vi "DAC freq and lock in test.vi"() -> ()   [LabVIEW 2012]
uses:
  <vilib>/Utility/file.llb/Read From Spreadsheet File (DBL).vi
  <vilib>/express/express arith-compare/Formula/XNode/ExpressFormulaBlockNode.xnode
panel:
  in  "resolution (1 Hz:1) 2":i32(ring)=1 items=["0.1 Hz", "1 Hz", "10 Hz", "100 Hz", "1 KHz", "10 KHz", "100 KHz", "1 MHz", "10 MHz", "100 MHz", "1 GHz"]
  in  "band (1-26.5 GHz:20) 2":i32(ring)=2
  in  "GPIB Address 2":string="19"
  in  "ODMR res file":path=path "C:/Users/Ouyang Group/Documents/Data/6-1-16/Dot 1 5mW local ODMR B freq min"
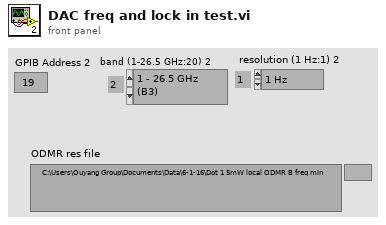
[diagram p1: front panel]
types:
  T1 = cluster{"source lock":bool, "lock frequency (Hz)":ext, "coarse tune":bool}
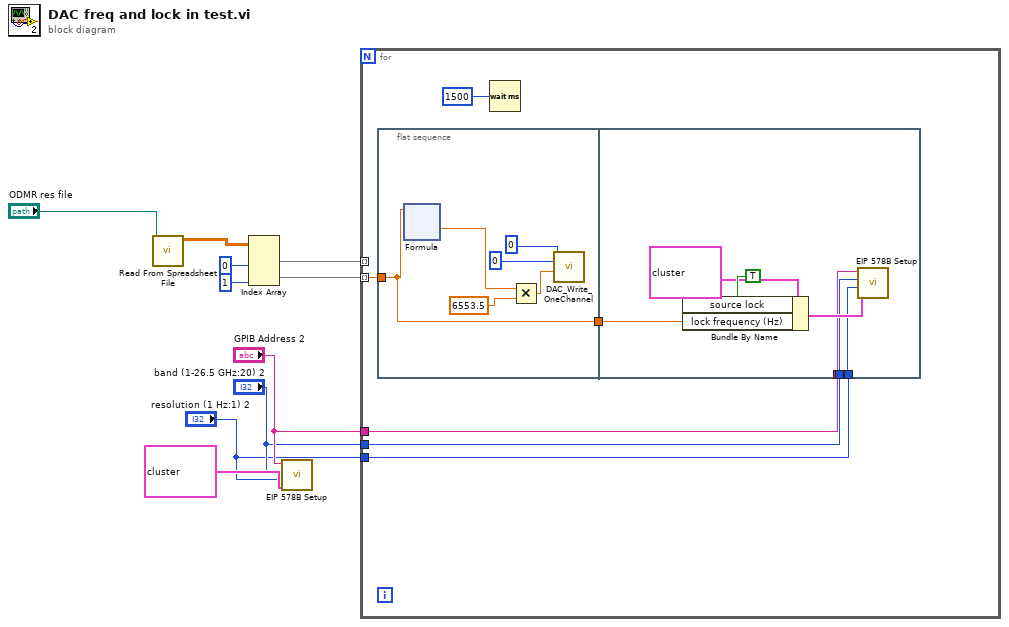
[diagram p0: block diagram]
diagram:
  n1 = call-poly <vilib>:"Read From Spreadsheet File.vi"("file path (dialog if empty)"="ODMR res file") -> ("all rows"=w9:dbl[][])  [unwired: 6 in, 4 out]
  n2 = Index Array(array=w9, index (col) #1=0 ("disabled index (col)"), index (col) #2=1 ("index (col)")) -> (element #1=w6:dbl[], element #2=w5:dbl[])  [unwired: 2 in]
  n3 = call "EIP 578B Setup.vi"("GPIB Address"="GPIB Address 2", "band (1-26.5 GHz:20)"="band (1-26.5 GHz:20) 2", "resolution (1 Hz:1)"="resolution (1 Hz:1) 2", "source locking"=T1 {"source lock"=FALSE, "lock frequency (Hz)"=1000000000.0, "coarse tune"=TRUE}) -> ()  [unwired: 2 in, 2 out]
  n4 = for {
    tunnel: w6 -> [_] mode=indexing
    tunnel: w5 -> [w16] mode=indexing
    tunnel: "GPIB Address 2" -> [w13]
    tunnel: "band (1-26.5 GHz:20) 2" -> [w12]
    tunnel: "resolution (1 Hz:1) 2" -> [w11]
    n5 = flat-sequence {
      tunnel: w16 -> [w17]
      tunnel: [w17] -> w14
      tunnel: w14 -> [w34]
      tunnel: w13 -> [w33]
      tunnel: w12 -> [w32]
      tunnel: w11 -> [w31]
      frame #0 {
        n6 = xnode "Formula"("X1"=w17) -> ("Result"=w18:dbl)  [unwired: 1 in, 1 out]
        n7 = Multiply(x=w18, y=6553.5) -> (x*y=w21:dbl)
        n8 = call "DAC_Write_OneChannel.vi"("Value"=w21, "Channel"=u16 0, "DeviceIndex"=u64 0) -> ()  [unwired: 7 in, 2 out]
      }
      frame #1 {
        n9 = Bundle By Name(cluster=T1 {"source lock"=FALSE, "lock frequency (Hz)"=1000000000.0, "coarse tune"=TRUE} ("source locking"), "source lock"=TRUE, "lock frequency (Hz)"=w34) -> (w36:T1)
        n10 = call "EIP 578B Setup.vi"("GPIB Address"=w33, "band (1-26.5 GHz:20)"=w32, "resolution (1 Hz:1)"=w31, "source locking"=w36) -> ()  [unwired: 2 in, 2 out]
      }
    }
    n11 = Wait (ms)(milliseconds to wait=u32 1500) -> ()  [unwired: 1 out]
  }
